vi "4channel-SHM.vi"() -> ()   [LabVIEW 2014]
doc: "Personal Daq 54 example.\nTriggering is immediate and readings are returned 1 scan at a time as available.\nBe sure to use the Acquisition Stop control for proper shutdown."
uses:
  <vilib>/Utility/error.llb/DialogType.ctl
  <vilib>/DAQmx/read.llb/DAQmx Read (Analog 1D DBL NChan 1Samp).vi
  <vilib>/Analysis/2dsp.llb/Complex FFT.vi
  <vilib>/DAQmx/create/channels.llb/DAQmx Create Channel (AI-Voltage-Basic).vi
  <vilib>/DAQmx/configure/timing.llb/DAQmx Timing (Sample Clock).vi
  <vilib>/DAQmx/miscellaneous.llb/DAQmx Fill In Error Info.vi
  <vilib>/measure/madcrms.llb/Basic Averaged DC-RMS for 1 Chan.vi
  <vilib>/express/express analysis/Spectral/Block/exnSpectralBlock spectral measurements peak poly.vi
  <vilib>/express/express analysis/Spectral/Block/exnSpectralBlock spectral measurements peak DDT.vi
  Instance           2 26Saved   noise_Nov07_2009_5 .vi
  Instance          18 26Saved   noise_Nov07_2009_5 .vi
  Instance           1 26Saved   noise_Nov07_2009_5 .vi
  Instance           4 26Saved   noise_Nov07_2009_5 .vi
  <vilib>/express/express analysis/Spectral/XNode/ExpressSpectralMeasurementsBlockNode.xnode
  <vilib>/measure/NI_MAPro.lvlib
  <vilib>/Analysis/NI_AALPro.lvlib
panel:
  out "Combined Spectrum 2":waveform(dbl)(graph)
  out "I/Q Spectrum 2":dynamicdata(graph)
  out "I/Q Signal 2":dynamicdata(graph)
  in  "Save Data":bool
  in  "Max. Heartrate":i32=90
  in  "Min. Heartrate":i32=50
  out "Heartrate":dbl
  out "max value 2":dbl
  in  "Max. Resp. Rate":i32=30
  in  "Min. Resp. Rate":i32=10
  out "Resp. Rate":dbl
  out "max value":dbl
  in  "input terminal configuration":i32(ring)=10083 items=["default"=-1, "RSE"=10083, "NRSE"=10078, "Differential"=10106, "Pseudodifferential"=12529]
  out "error out":errorcluster
  in  "stop":bool
  in  "Maximum Value":dbl=5.0 format="%0.2f"
  in  "Minimum Value":dbl=-2.0 format="%0.2f"
  in  "Rate":dbl=20.0 caption="Sample Rate (Hz)" format="%0.2f"
  in  "Samples per Channel":i32=1
  out "Combined Spectrum":waveform(dbl)(graph)
  out "I/Q Spectrum":dynamicdata(graph)
  out "Respiration Q":dbl=19.665142208058892 format="%#_3g"
  out "Respiration I":dbl=19.7 format="%#_3g"
  in  "FFT":i32=256
  out "I/Q Signal":dynamicdata(graph)
  in  "t0":timestamp=timestamp(3198752888.296 s since 1904-01-01)
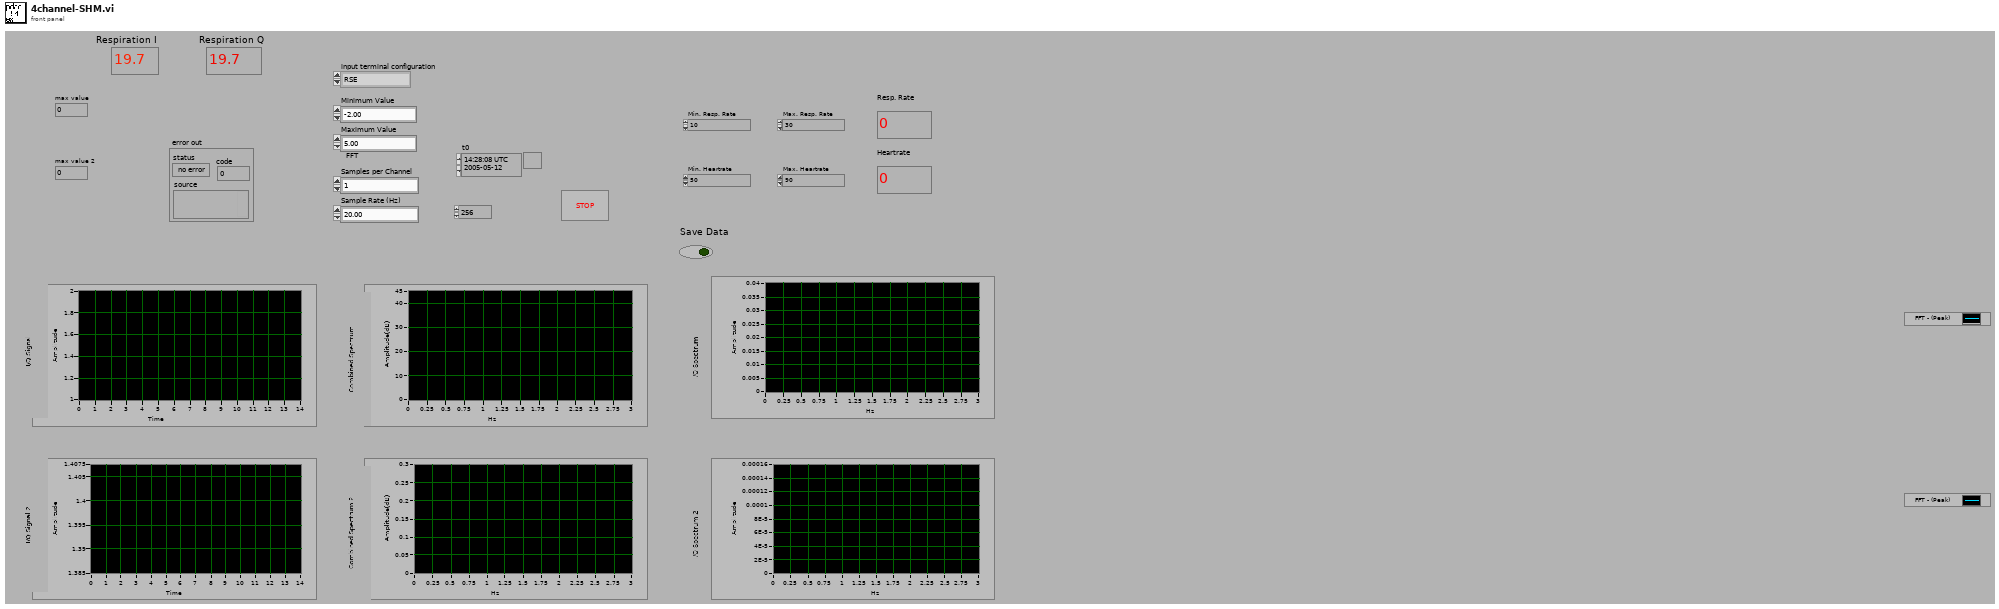
[diagram p1: front panel]
types:
  T1 = typedef "DialogType.ctl" = u16
  T2 = cluster{"averaging mode":u16, "weighting mode":u16, "number of averages":u32}
  T3 = cluster{"dB On (F)":bool, "unwrap phase (F)":bool, "convert to degree (F)":bool}
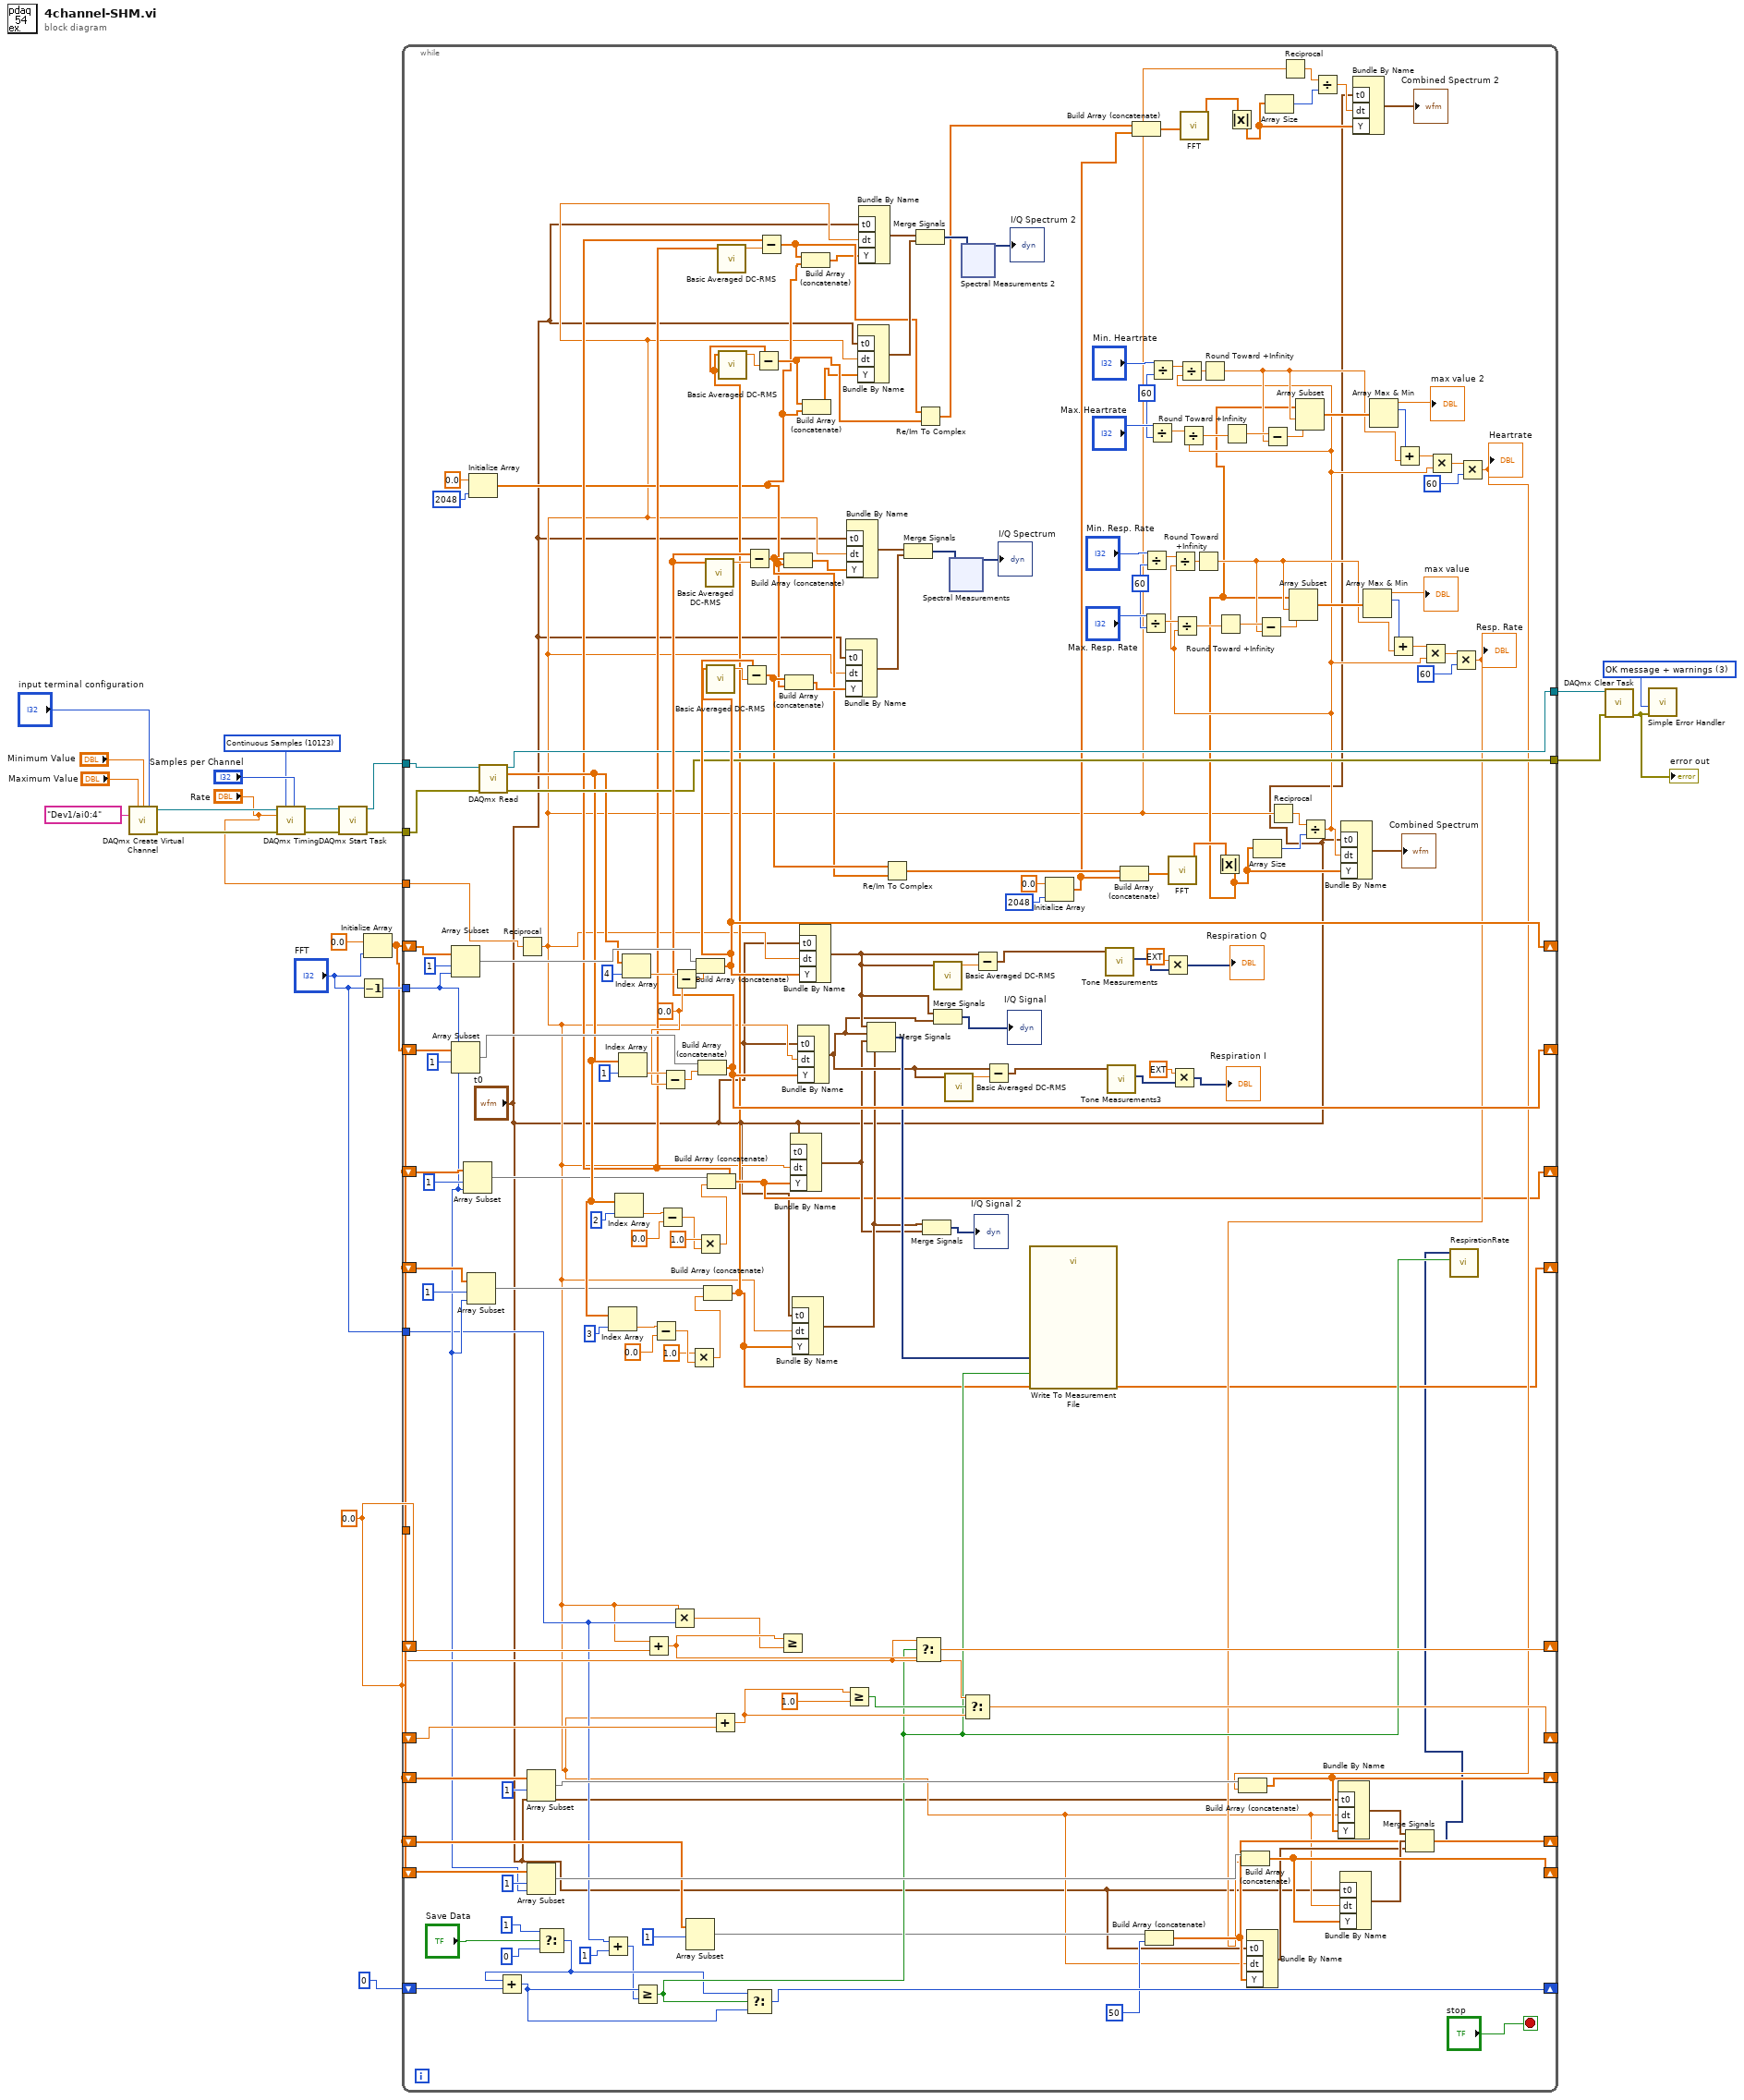
[diagram p0: block diagram]
diagram:
  w3 = 0.0 ("element")
  w9 = T1 3 items=["no dialog", "OK message", "continue or stop message", "OK message + warnings", "continue/stop + warnings"] ("type of dialog (OK msg:1)")
  w16 = 10123 items=["Finite Samples"=10178, "Continuous Samples"=10123] ("sample mode")
  n1 = call-poly <vilib>:"DAQmx Create Virtual Channel.vi"("maximum value"="Maximum Value", "minimum value"="Minimum Value", "input terminal configuration"="input terminal configuration", "physical channels"=tag "Dev1/ai0:4") -> ("task out"=w17:refnum<k21>, "error out"=w19:errorcluster)  [unwired: 5 in, 5 out]
  n2 = call-poly <vilib>:"DAQmx Timing.vi"("task/channels in"=w17, "sample mode"=w16, "samples per channel"="Samples per Channel", "rate"="Rate", "error in"=w19) -> ("task out"=w15:refnum<k21>, "error out"=w14:errorcluster)  [unwired: 2 in, 7 out]
  n3 = call <vilib>:"DAQmx Start Task.vi"("task/channels in"=w15, "error in"=w14) -> ("task out"=w12:refnum<k21>, "error out"=w11:errorcluster)  [unwired: 12 out]
  n4 = Decrement(x="FFT") -> (x-1=w22:i32)
  n5 = Initialize Array(0.0 ("element"), "FFT") -> (w1:dbl[])
  n6 = while {
    shift-right: [w167] -> _
    shift-left: w1 -> [w198]
    tunnel: w22 -> [w67]
    shift-right: [w166] -> _
    shift-left: w1 -> [w189]
    tunnel: w12 -> [w165]
    tunnel: w11 -> [w164]
    tunnel: "Rate" -> [w163]
    tunnel: [w162] -> w8
    tunnel: [w161] -> w7
    shift-right: [w154] -> _
    shift-left: w3 -> [w152]
    tunnel: "FFT" -> [w51]
    tunnel: w3 -> [w146]
    shift-right: [w150] -> _
    shift-left: w3 -> [w147]
    shift-right: [w132] -> _
    shift-left: w1 -> [w140]
    shift-right: [w133] -> _
    shift-left: w1 -> [w136]
    shift-right: [w91] -> _
    shift-left: 0 -> [w93]
    shift-right: [w42] -> _
    shift-left: w1 -> [w84]
    shift-right: [w75] -> _
    shift-left: w1 -> [w79]
    shift-right: [w41] -> _
    shift-left: w1 -> [w69]
    stop <- "stop" stop-if-true
    w96 = 60
    w112 = 60
    w183 = 0.0 ("element")
    n7 = Array Subset(array=w198, index=1, length=w67) -> (w196:dbl[])
    n8 = Array Subset(array=w189, index=1, length=w67) -> (w187:dbl[])
    n9 = Array Subset(array=w84, index=1, length=w67) -> (w43:dbl[])
    n10 = Array Subset(array=w69, index=1, length=w67) -> (w59:dbl[])
    n11 = Initialize Array(0.0 ("element"), 2048 ("dimension size")) -> (w38:dbl[])
    n12 = call-poly <vilib>:"DAQmx Read.vi"("task/channels in"=w165, "error in"=w164) -> ("task out"=w162:refnum<k21>, "data"=w60:dbl[], "error out"=w161:errorcluster)  [unwired: 11 out]
    n13 = Reciprocal(x=w163) -> (1/x=w26:dbl)
    n14 = Array Subset(array=w136, index=1) -> (w135:dbl[])  [unwired: 1 in]
    n15 = Array Subset(array=w140, index=1, length=w67) -> (w139:dbl[])
    n16 = Select(t=1, s="Save Data", f=0) -> (s? t:f=w87:i32)
    n17 = Add(x=w87, y=w93) -> (x+y=w92:i32)
    n18 = Add(x=w51, y=1 ("index")) -> (x+y=w50:i32)
    n19 = Index Array(array=w60, index=3 ("index (row)")) -> (element=w63:dbl)
    n20 = Index Array(array=w60, index=2 ("index (row)")) -> (element=w81:dbl)
    n21 = Index Array(array=w60, index=1 ("index (row)")) -> (element=w184:dbl)
    n22 = Index Array(array=w60, index=4 ("index (row)")) -> (element=w185:dbl)
    n23 = Greater Or Equal?(x=w92, y=w50) -> (x >= y?=w90:bool)
    n24 = Add(x=w26, y=w152) -> (x+y=w155:dbl)
    n25 = Subtract(x=w63, y=0.0 ("element")) -> (x-y=w66:dbl)
    n26 = Subtract(x=w81, y=0.0 ("element")) -> (x-y=w71:dbl)
    n27 = Subtract(x=w184, y=w183) -> (x-y=w177:dbl)
    n28 = Multiply(x=w26, y=w51) -> (x*y=w153:dbl)
    n29 = Subtract(x=w185, y=w183) -> (x-y=w178:dbl)
    n30 = Array Subset(array=w79, index=1) -> (w77:dbl[])  [unwired: 1 in]
    n31 = Multiply(x=1.0, y=w66) -> (x*y=w61:dbl)
    n32 = Build Array (concatenate)(w196, w178) -> (w167:dbl[])
    n33 = Multiply(x=1.0, y=w71) -> (x*y=w70:dbl)
    n34 = Build Array (concatenate)(w187, w177) -> (w166:dbl[])
    n35 = Build Array (concatenate)(w59, w61) -> (w41:dbl[])
    n36 = call-poly <vilib>:"Basic Averaged DC-RMS.vi"("signal in"=w166) -> ("DC value"=w176:dbl)  [unwired: 4 in, 6 out]
    n37 = call-poly <vilib>:"Basic Averaged DC-RMS.vi"("signal in"=w167) -> ("DC value"=w175:dbl)  [unwired: 4 in, 6 out]
    n38 = Build Array (concatenate)(w43, w70) -> (w42:dbl[])
    n39 = Add(x=w26, y=w147) -> (x+y=w151:dbl)
    n40 = call-poly <vilib>:"Basic Averaged DC-RMS.vi"("signal in"=w42) -> ("DC value"=w44:dbl)  [unwired: 4 in, 6 out]
    n41 = call-poly <vilib>:"Basic Averaged DC-RMS.vi"("signal in"=w41) -> ("DC value"=w45:dbl)  [unwired: 4 in, 6 out]
    n42 = Subtract(x=w167, y=w175) -> (x-y=w157:dbl[])
    n43 = Subtract(x=w166, y=w176) -> (x-y=w156:dbl[])
    n44 = Select(t=w87, s=w90, f=w92) -> (s? t:f=w91:i32)
    n45 = Subtract(x=w41, y=w45) -> (x-y=w40:dbl[])
    n46 = Subtract(x=w42, y=w44) -> (x-y=w37:dbl[])
    n47 = Greater Or Equal?(x=w155, y=w153) -> ()  [unwired: 1 out]
    n48 = Build Array (concatenate)(w156, w38) -> (w181:dbl[])
    n49 = Build Array (concatenate)(w157, w38) -> (w182:dbl[])
    n50 = Bundle By Name("t0"="t0", "dt"=w26, "Y"=w42) -> (w53:waveform(dbl))  [unwired: 1 out]
    n51 = Bundle By Name("t0"="t0", "dt"=w26, "Y"=w41) -> (w54:waveform(dbl))  [unwired: 1 out]
    n52 = Bundle By Name("t0"="t0", "dt"=w26, "Y"=w166) -> (w56:waveform(dbl))  [unwired: 1 out]
    n53 = Bundle By Name("t0"="t0", "dt"=w26, "Y"=w167) -> (w57:waveform(dbl))  [unwired: 1 out]
    n54 = Build Array (concatenate)(w37, w38) -> (w36:dbl[])
    n55 = Build Array (concatenate)(w40, w38) -> (w39:dbl[])
    n56 = Greater Or Equal?(x=w151, y=1.0) -> (x >= y?=w148:bool)
    n57 = Bundle By Name("t0"="t0", "dt"=w26, "Y"=w182) -> (w172:waveform(dbl))  [unwired: 1 out]
    n58 = Bundle By Name("t0"="t0", "dt"=w26, "Y"=w181) -> (w173:waveform(dbl))  [unwired: 1 out]
    n59 = Bundle By Name("t0"="t0", "dt"=w26, "Y"=w39) -> (w48:waveform(dbl))  [unwired: 1 out]
    n60 = Bundle By Name("t0"="t0", "dt"=w26, "Y"=w36) -> (w47:waveform(dbl))  [unwired: 1 out]
    n61 = Merge Signals(w57, w56, w53, w54) -> (w158:dynamicdata)
    n62 = Re/Im To Complex(1:w156, 2:w157) -> (0:w179:cdb[])
    n63 = Merge Signals(w173, w172) -> (w174:dynamicdata)
    n64 = Select(t=w146, s=w90, f=w155) -> (s? t:f=w154:dbl)
    n65 = Merge Signals(w47, w48) -> (w46:dynamicdata)
    n66 = Re/Im To Complex(1:w40, 2:w37) -> (0:w27:cdb[])
    n67 = Merge Signals(w54, w53) -> (→"I/Q Signal 2":dynamicdata)
    n68 = call-poly <vilib>:"Basic Averaged DC-RMS.vi"("signal in"=w57) -> ("DC value"=w145:dbl)  [unwired: 4 in, 6 out]
    n69 = Merge Signals(w57, w56) -> (→"I/Q Signal":dynamicdata)
    n70 = call-poly <vilib>:"Basic Averaged DC-RMS.vi"("signal in"=w56) -> ("DC value"=w143:dbl)  [unwired: 4 in, 6 out]
    n71 = xnode "Spectral Measurements"("Signals"=w174) -> ("FFT - (Peak)"=→"I/Q Spectrum":dynamicdata)  [unwired: 2 in, 3 out]
    n72 = xnode "Spectral Measurements 2"("Signals"=w46) -> ("FFT - (Peak)"=→"I/Q Spectrum 2":dynamicdata)  [unwired: 2 in, 3 out]
    n73 = Select(t=w146, s=w148, f=w151) -> (s? t:f=w150:dbl)
    n74 = Subtract(x=w57, y=w145) -> (x-y=w144:waveform(dbl))
    n75 = Subtract(x=w56, y=w143) -> (x-y=w142:waveform(dbl))
    n76 = call "Write To Measurement File"("Signals"=w158, "Enable"=w90) -> ()  [unwired: 5 in, 13 out]
    n77 = Initialize Array(0.0 ("element"), 2048 ("dimension size")) -> (w28:dbl[])
    n78 = call "Tone Measurements"("Signals"=w144) -> ("Frequency"=w193:dynamicdata)  [unwired: 1 in, 9 out]
    n79 = call "Tone Measurements3"("Signals"=w142) -> ("Frequency"=w190:dynamicdata)  [unwired: 1 in, 9 out]
    n80 = Build Array (concatenate)(w179, w28) -> (w168:cdb[])
    n81 = Build Array (concatenate)(w27, w28) -> (w31:cdb[])
    n82 = Divide(x="Max. Resp. Rate", y=w112) -> (x/y=w127:dbl)
    n83 = Divide(x="Min. Resp. Rate", y=w112) -> (x/y=w128:dbl)
    n84 = Build Array (concatenate)(w77, 50 ("index")) -> (w75:dbl[])
    n85 = Divide(x="Max. Heartrate", y=w96) -> (x/y=w110:dbl)
    n86 = Divide(x="Min. Heartrate", y=w96) -> (x/y=w111:dbl)
    n87 = Multiply(x=ext 60.0, y=w193) -> (x*y=→"Respiration Q":dynamicdata)
    n88 = call-poly <vilib>:"FFT.vi"("X"=w168) -> ("FFT {X}"=w171:cdb[])  [unwired: 2 in, 8 out]
    n89 = Multiply(x=ext 60.0, y=w190) -> (x*y=→"Respiration I":dynamicdata)
    n90 = call-poly <vilib>:"FFT.vi"("X"=w31) -> ("FFT {X}"=w29:cdb[])  [unwired: 2 in, 8 out]
    n91 = Absolute Value(x=w171) -> (abs(x)=w85:dbl[])
    n92 = Absolute Value(x=w29) -> (abs(x)=w35:dbl[])
    n93 = Bundle By Name("t0"="t0", "dt"=w26, "Y"=w75) -> (w76:waveform(dbl))  [unwired: 1 out]
    n94 = Array Size(array=w85) -> (size(s)=w169:i32)
    n95 = Array Size(array=w35) -> (size(s)=w30:i32)
    n96 = Reciprocal(x=w26) -> (1/x=w115:dbl)
    n97 = Reciprocal(x=w26) -> (1/x=w33:dbl)
    n98 = Divide(x=w115, y=w169) -> (x/y=w95:dbl)
    n99 = Divide(x=w128, y=w95) -> (x/y=w126:dbl)
    n100 = Divide(x=w127, y=w95) -> (x/y=w125:dbl)
    n101 = Divide(x=w111, y=w95) -> (x/y=w109:dbl)
    n102 = Divide(x=w110, y=w95) -> (x/y=w108:dbl)
    n103 = Round Toward +Infinity(x=w126) -> (ceil(x): smallest int >= x=w119:dbl)
    n104 = Round Toward +Infinity(x=w109) -> (ceil(x): smallest int >= x=w102:dbl)
    n105 = Round Toward +Infinity(x=w125) -> (ceil(x): smallest int >= x=w123:dbl)
    n106 = Round Toward +Infinity(x=w108) -> (ceil(x): smallest int >= x=w106:dbl)
    n107 = Subtract(x=w123, y=w119) -> (x-y=w124:dbl)
    n108 = Subtract(x=w106, y=w102) -> (x-y=w107:dbl)
    n109 = Array Subset(array=w85, index=w119, length=w124) -> (w122:dbl[])
    n110 = Array Subset(array=w85, index=w102, length=w107) -> (w105:dbl[])
    n111 = Divide(x=w33, y=w30) -> (x/y=w34:dbl)
    n112 = Bundle By Name("t0"="t0", "dt"=w95, "Y"=w85) -> (→"Combined Spectrum":waveform(dbl))  [unwired: 1 out]
    n113 = Bundle By Name("t0"="t0", "dt"=w34, "Y"=w35) -> (→"Combined Spectrum 2":waveform(dbl))  [unwired: 1 out]
    n114 = Array Max & Min(array=w122) -> (max value=→"max value":dbl, max index (indices)=w120:i32)  [unwired: 2 out]
    n115 = Array Max & Min(array=w105) -> (max value=→"max value 2":dbl, max index (indices)=w103:i32)  [unwired: 2 out]
    n116 = Add(x=w120, y=w119) -> (x+y=w118:dbl)
    n117 = Add(x=w103, y=w102) -> (x+y=w101:dbl)
    n118 = Multiply(x=w118, y=w95) -> (x*y=w117:dbl)
    n119 = Multiply(x=w101, y=w95) -> (x*y=w100:dbl)
    n120 = Multiply(x=w117, y=60) -> (x*y=w74:dbl)
    "Resp. Rate" <- w74
    n121 = Build Array (concatenate)(w139, w74) -> (w132:dbl[])
    n122 = Bundle By Name("t0"="t0", "dt"=w26, "Y"=w132) -> (w130:waveform(dbl))  [unwired: 1 out]
    n123 = Multiply(x=w100, y=60) -> (x*y=w94:dbl)
    "Heartrate" <- w94
    n124 = Build Array (concatenate)(w135, w94) -> (w133:dbl[])
    n125 = Bundle By Name("t0"="t0", "dt"=w26, "Y"=w133) -> (w131:waveform(dbl))  [unwired: 1 out]
    n126 = Merge Signals(w131, w130, w76) -> (w24:dynamicdata)
    n127 = call "RespirationRate"("Enable"=w90, "Signals"=w24) -> ()  [unwired: 3 in, 7 out]
  }
  n128 = call <vilib>:"DAQmx Clear Task.vi"("task in"=w8, "error in"=w7) -> ("error out"=w6:errorcluster)  [unwired: 13 out]
  "error out" <- w6
  n129 = call <vilib>:"Simple Error Handler.vi"("type of dialog (OK msg:1)"=w9, "error in (no error)"=w6) -> ()  [unwired: 8 out]
